vi "LM fitting parameter assignment.vi"(10 "Parameter array":T2(array[cluster])=[{"initial param"=1.0, "variable?"=TRUE, "lower limit"=0.0, "upper limit"=0.0, "name"="a0"}, {"initial param"=2.0, "variable?"=TRUE, "lower limit"=0.0, "upper limit"=0.0, "name"="a1"}, {"initial param"=3.0, "variable?"=TRUE, "lower limit"=0.0, "upper limit"=0.0, "name"="c"}, {"initial param"=4.0, "variable?"=TRUE, "lower limit"=0.0, "upper limit"=0.0, "name"="tau"}, {"initial param"=5.0, "variable?"=TRUE, "lower limit"=0.0, "upper limit"=0.0, "name"="b"}], 11 "Fitting Function (write with ai's)":string="a0+a1*x^(-c)*exp(-(tau/x)^b)") -> (0 "boolean array":bool[](array[boolean]), 1 "initial initial":dbl[](array[numeric]), 2 "initial parameters":dbl[](array[numeric])=[1.0, 2.0, 3.0, 4.0, 5.0], 3 "Output for LM fitting":T1={"model"="a0+a1*x^(-c)*exp(-(tau/x)^b)", "Parameters"=["a0", "a1", "c", "tau", "b"], "x"="x"})   [LabVIEW 2020]
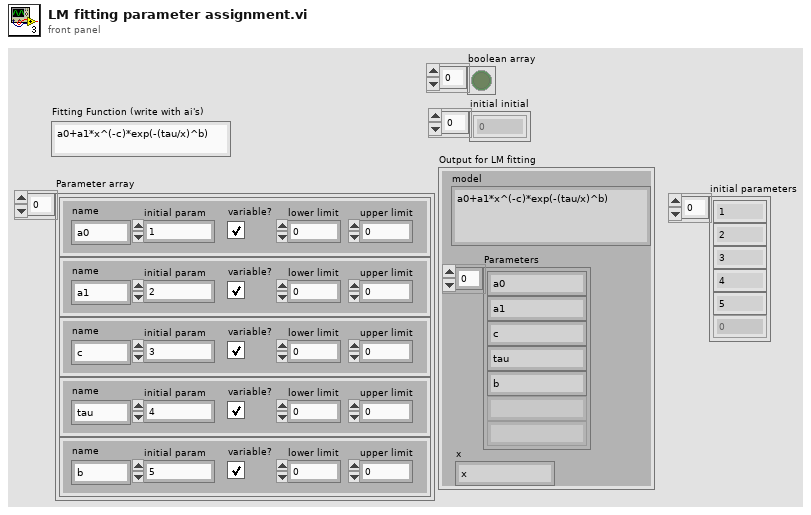
[diagram p1: front panel]
types:
  T1 = cluster{"model":string, "Parameters":string[], "x":string}
  T2 = cluster{"initial param":dbl, "variable?":bool, "lower limit":dbl, "upper limit":dbl, "name":string}[]
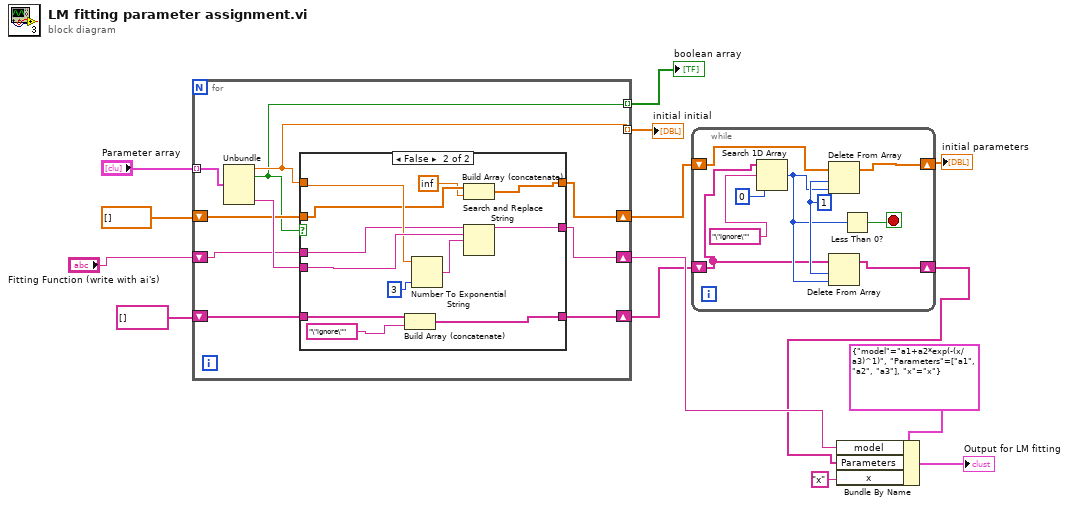
[diagram p0: block diagram]
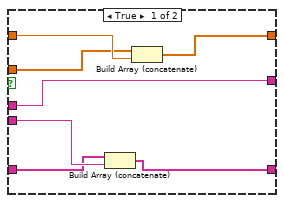
[diagram p2: hidden frame]
diagram:
  n1 = for {
    tunnel: "Parameter array" -> [w24] mode=indexing
    shift-right: [w21] -> w11
    shift-left: "Fitting Function (write with ai's)" -> [w22]
    shift-right: [w19] -> w4
    shift-left: string[] [] ("appended array") -> [w20]
    shift-right: [w17] -> w6
    shift-left: dbl[] [] ("appended array") -> [w18]
    tunnel: [w16] -> w1 mode=indexing
    tunnel: [w15] -> w2 mode=indexing
    n2 = Unbundle(w24) -> ("initial param"=w16:dbl, "variable?"=w15:bool, "name"=w23:string)  [unwired: 2 out]
    n3 = case shown="False" w15 {
      tunnel: w16 -> [w27 w41]
      tunnel: w23 -> [w30 w43]
      tunnel: [w31 w42] -> w21
      tunnel: [w25 w32] -> w17
      tunnel: w22 -> [w31 w38]
      tunnel: w20 -> [w29 w37]
      tunnel: [w28 w36] -> w19
      tunnel: w18 -> [w26 w34]
      frame True {
        n4 = Build Array (concatenate)(w29, w30) -> (w28:string[])
        n5 = Build Array (concatenate)(w26, w27) -> (w25:dbl[])
      }
      frame False {
        n6 = Build Array (concatenate)(w37, "\"ignore\"" ("name")) -> (w36:string[])
        n7 = Number To Exponential String(number=w41, precision (6)=i16 3) -> (E-format string=w40:string)  [unwired: 2 in]
        n8 = Build Array (concatenate)(w34, inf ("initial param")) -> (w32:dbl[])
        n9 = Search and Replace String(input string=w38, search string=w43, replace string=w40) -> (result string=w42:string)  [unwired: 5 in, 3 out]
      }
    }
  }
  "boolean array" <- w2
  "initial initial" <- w1
  n10 = while {
    shift-right: [w51] -> w5
    shift-left: w6 -> [w47]
    shift-right: [w44] -> w3
    shift-left: w4 -> [w45]
    stop <- w50 stop-if-true
    w49 = 1 ("length")
    n11 = Search 1D Array(1D array=w45, element="\"ignore\"" ("name"), start index (0)=0) -> (index of element=w48:i32)
    n12 = Delete From Array(array=w47, length=w49, index=w48) -> (array with subset deleted=w51:dbl[])  [unwired: 1 out]
    n13 = Delete From Array(array=w45, length=w49, index=w48) -> (array with subset deleted=w44:string[])  [unwired: 1 out]
    n14 = Less Than 0?(x=w48) -> (x < 0?=w50:bool)
  }
  "initial parameters" <- w5
  n15 = Bundle By Name(cluster=T1 {"model"="a1+a2*exp(-(x/a3)^1)", "Parameters"=["a1", "a2", "a3"], "x"="x"} ("model description"), "model"=w11, "Parameters"=w3, "x"="x") -> (→"Output for LM fitting":T1)
